vi "RunningVIsChange.vi"(2 "error in (no error)":errorcluster, 3 "newstate":bool, 4 "name":string) -> (0 "error out":errorcluster, 1 "JSON Tree out (JSON Object)":variant)   [LabVIEW 2018]
uses:
  <vilib>/LVH/i3 JSON/JSON Generation/Create Value Files/Create Value - Object.vi
  <vilib>/LVH/i3 JSON/JSON Generation/Add Object Parameter Files/Add Object Parameter - String.vi
  <vilib>/LVH/i3 JSON/JSON Generation/Add Object Parameter Files/Add Object Parameter - Boolean.vi
  <vilib>/LVH/i3 JSON/i3-json.lvlib
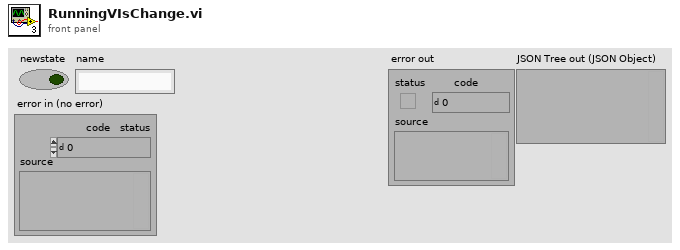
[diagram p1: front panel]
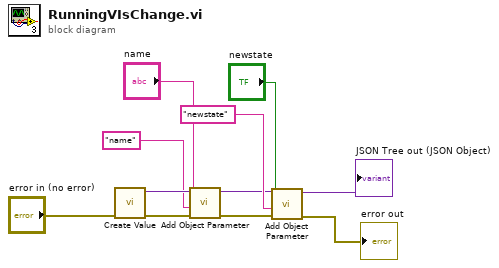
[diagram p0: block diagram]
diagram:
  n1 = call-poly <vilib>:"Create Value.vi"("error in (no error)"="error in (no error)") -> ("error out"=w6:errorcluster, "JSON Tree"=w9:variant)  [unwired: 9 in]
  n2 = call-poly <vilib>:"Add Object Parameter.vi"("error in (no error)"=w6, "Name"="name", "String"="name", "JSON Tree in (JSON Object)"=w9) -> ("error out"=w7:errorcluster, "JSON Tree out (JSON Object)"=w8:variant)  [unwired: 6 in]
  n3 = call-poly <vilib>:"Add Object Parameter.vi"("error in (no error)"=w7, "Name"="newstate", "Boolean"="newstate", "JSON Tree in (JSON Object)"=w8) -> ("error out"=→"error out":errorcluster, "JSON Tree out (JSON Object)"=→"JSON Tree out (JSON Object)":variant)  [unwired: 6 in]
